vi "Set From File.vi"(8 "error in (no error)":errorcluster, 10 "Memory binary":path, 11 "Memory in":refnum<class "Memory.lvclass">) -> (0 "error out":errorcluster, 3 "Memory out":refnum<class "Memory.lvclass">)   [LabVIEW 2021, in "Memory.lvclass"]
uses:
  Memory.lvclass
  Memory.lvclass/Memory.ctl
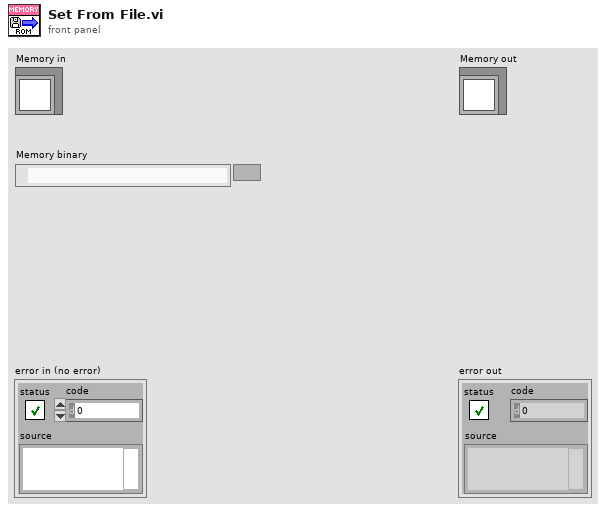
[diagram p1: front panel]
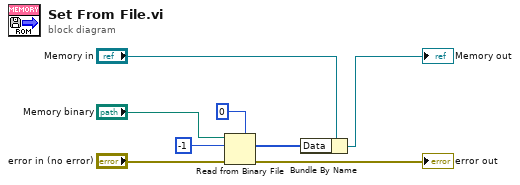
[diagram p0: block diagram]
diagram:
  n1 = Read from Binary File(5:u8 0, 8:"error in (no error)", 10:-1 ("count (1)"), 11:"Memory binary") -> (0:→"error out":errorcluster, 2:w1:u8[])  [unwired: 2 in, 2 out]
  n2 = Bundle By Name(cluster="Memory in", "Data"=w1) -> (→"Memory out":refnum<class "Memory.lvclass">)
